vi "Initialize.vi"(6 "Serial Configuration":T1={"Baud Rate"=9600, "Parity"=0, "Data Bits"=8, "Stop Bits"=10, "Flow Control"=0} {"Flow Control" items=["None", "XON/XOFF", "RTS/CTS", "XON/XOFF & RTS/CTS", "DTR/DSR", "XON/XOFF & DTR/DSR"]; "Stop Bits" items=["1.0"=10, "1.5"=15, "2.0"=20]; "Data Bits" items=["7"=7, "8"=8]; "Parity" items=["None", "Odd", "Even", "Mark", "Space"]; "Baud Rate" items=["300"=300, "600"=600, "1200"=1200, "2400"=2400, "4800"=4800, "9600"=9600, "19200"=19200]}, 7 "error in (no error)":errorcluster, 8 "ID Query (T: Check)":bool=TRUE, 9 "VISA resource name":refnum<visa-resource-name>="TCPIP0::169.254.213.32::inst0::INSTR", 10 "BH Druck PACE Series in":refnum<class "BH Druck PACE Series.lvclass">) -> (0 "error out":errorcluster, 3 "BH Druck PACE Series out":refnum<class "BH Druck PACE Series.lvclass">)   [LabVIEW 2022 SP3, in "BH Druck PACE Series.lvclass"]
uses:
  BH Druck PACE Series.lvclass
  BH Druck PACE Series.lvclass/BH Druck PACE Series.ctl
panel:
  out "VISA resource name out":refnum<visa-resource-name>
  # "2010-2022 BH Druck Ltd.  ALL RIGHTS RESERVED."
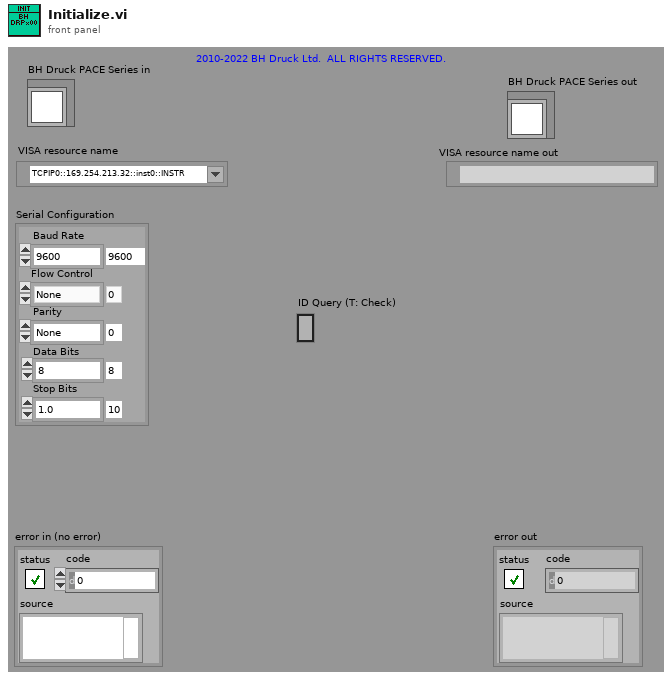
[diagram p1: front panel]
types:
  T1 = cluster{"Baud Rate":u32, "Parity":u16, "Data Bits":u16, "Stop Bits":u16, "Flow Control":u16}
  T2 = cluster{"status":bool, "code":i32, "VI name":string}
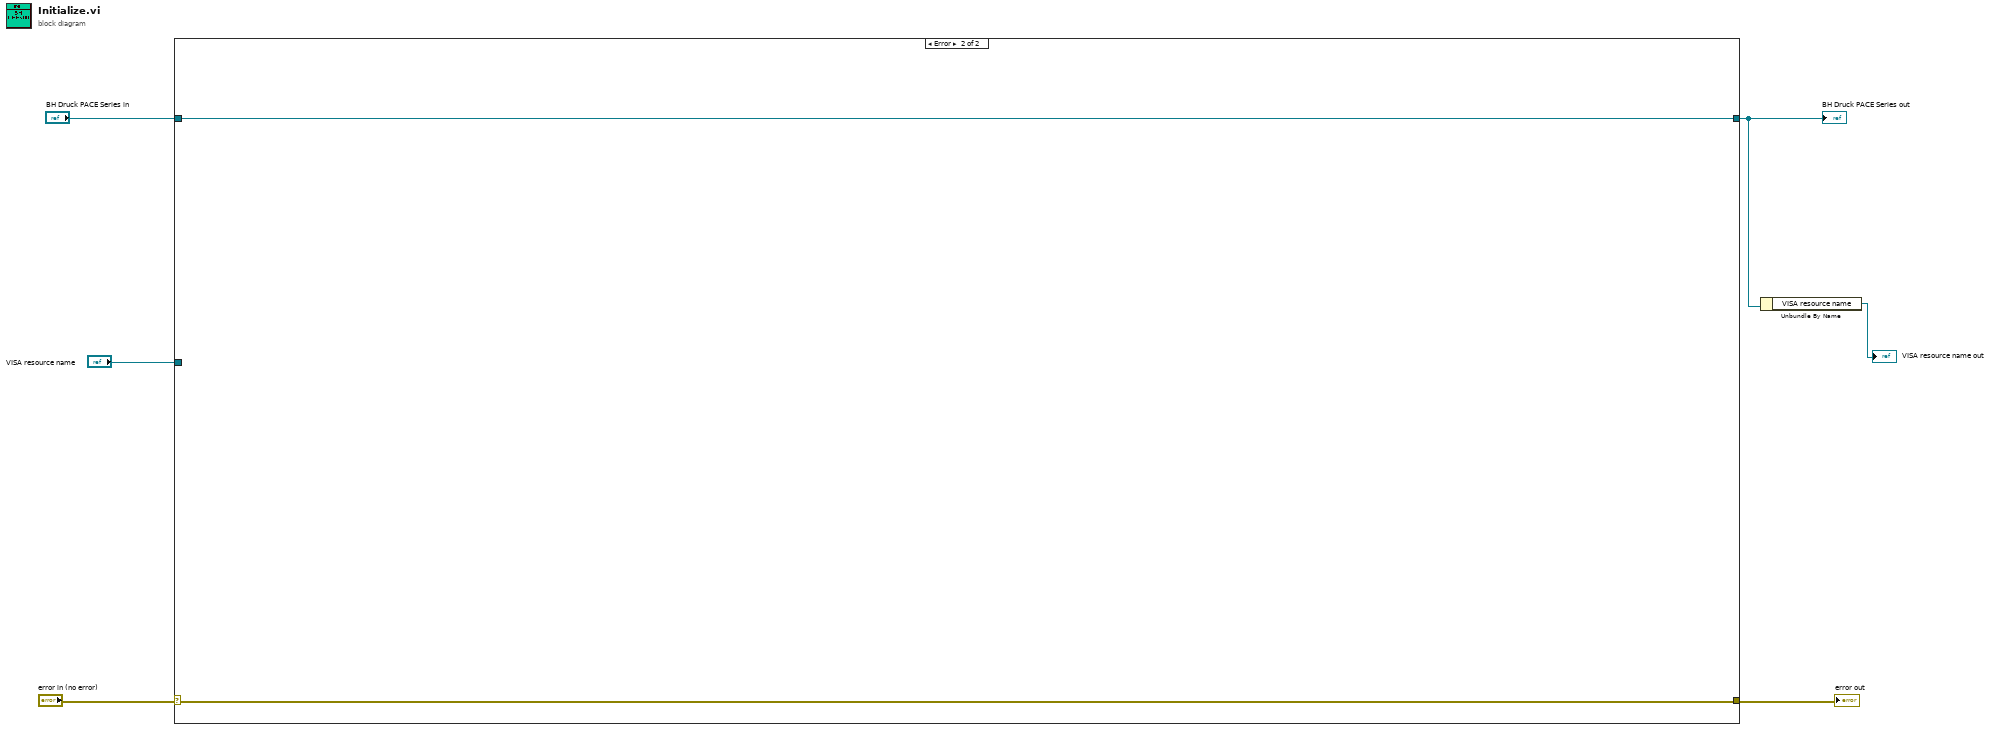
[diagram p0: block diagram]
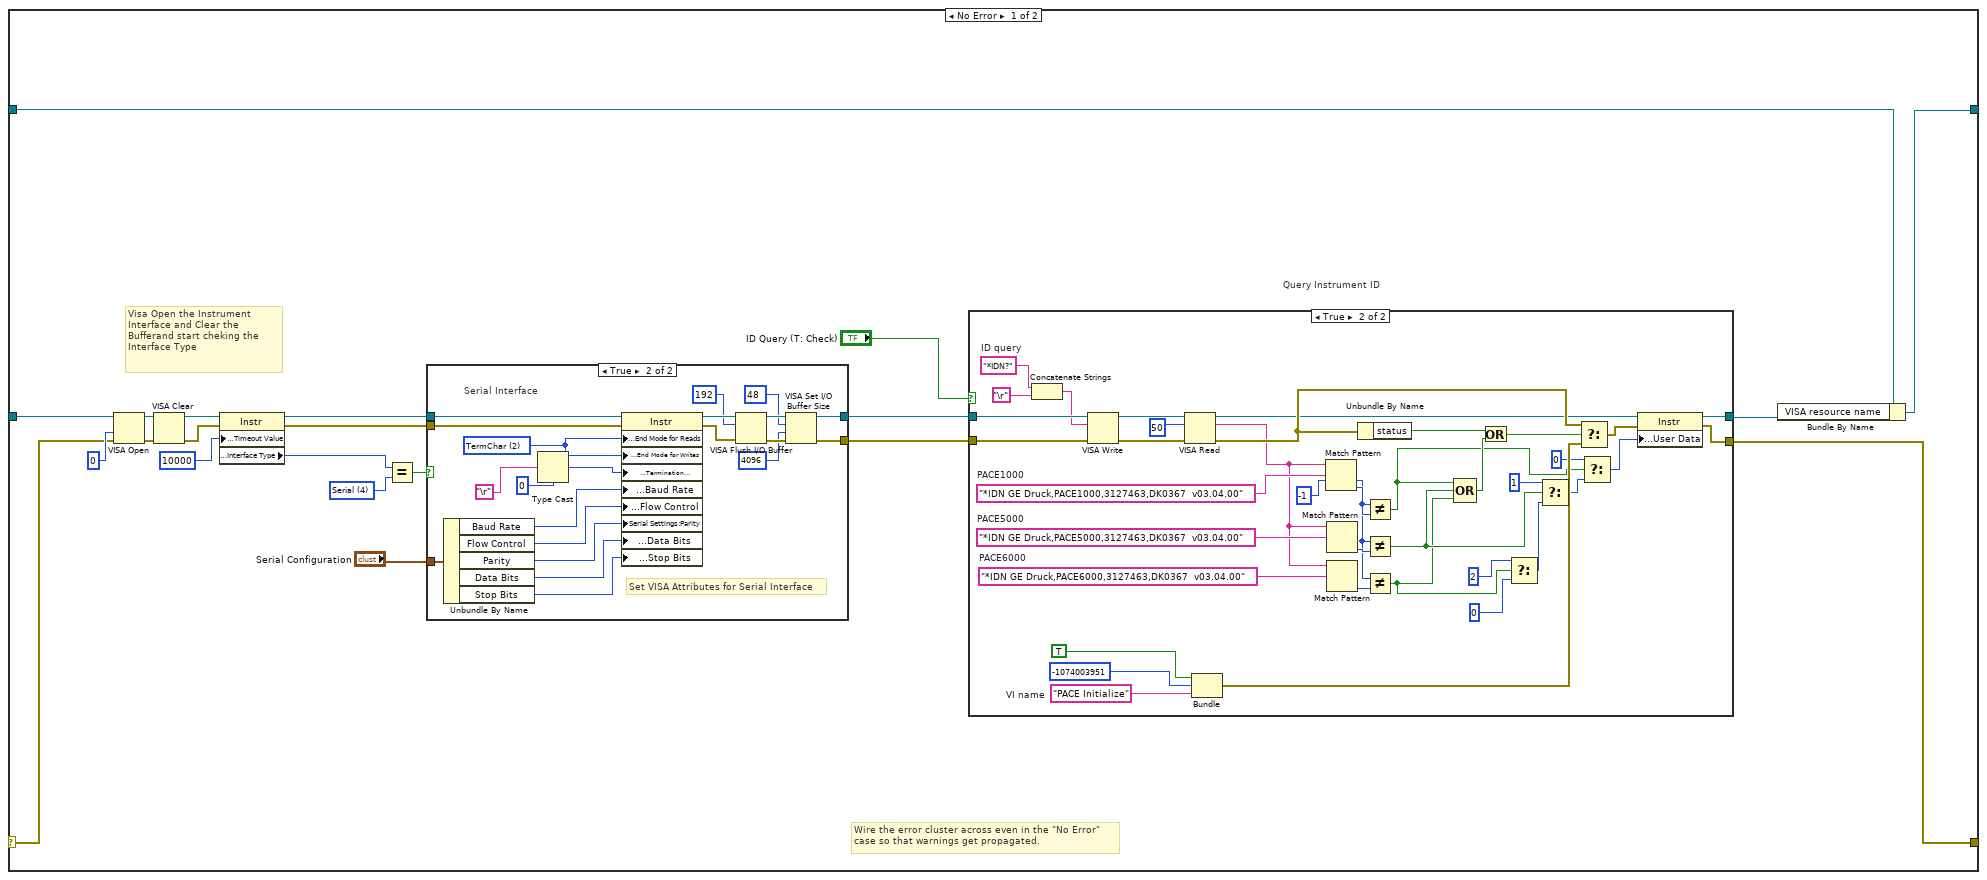
[diagram p2: hidden frame]
diagram:
  n1 = case shown="Error" "error in (no error)" {
    selector: "error in (no error)" -> [w15 w92]
    tunnel: [w8 w92] -> w5
    tunnel: [w7 w91] -> w2
    tunnel: "BH Druck PACE Series in" -> [w14 w91]
    tunnel: "VISA resource name" -> [w13 _]
    frame No Error {
      w22 = u16 4 items=["GPIB"=1, "VXI"=2, "GPIB-VXI"=3, "Serial"=4, "PXI"=5, "TCPIP"=6, "USB"=7] ("Interface Information:Interface Type")
      # "Visa Open the Instrument  Interface and Clear the Bufferand start cheking the \nInterface Type"
      # "Query Instrument ID"
      # "Wire the error cluster across even in the \"No Error\"\ncase so that warnings get propagated."
      n2 = VISA Open(access mode=u32 0, error in (no error)=w15, VISA resource name=w13) -> (VISA resource name=w20:refnum<visa-resource-name>, error out=w19:errorcluster)  [unwired: 2 in]
      n3 = VISA Clear(VISA resource name=w20, error in (no error)=w19) -> (VISA resource name out=w18:refnum<visa-resource-name>, error out=w17:errorcluster)
      n4 = property on="Property Node" class="Instr"(reference=w18, error in=w17, "General Settings:Timeout Value"=u32 10000) -> (reference out=w25:refnum<visa-resource-name>, error out=w24:errorcluster, "Interface Information:Interface Type"=w27:u16)
      n5 = Equal?(x=w27, y=w22) -> (x = y?=w23:bool)
      n6 = case shown="True" w23 {
        tunnel: [w68 w87] -> w11
        tunnel: [w69 w84] -> w10
        tunnel: w25 -> [w68 w89]
        tunnel: w24 -> [w69 w90]
        tunnel: "Serial Configuration" -> [_ w71]
        frame False {
          # "This Case Executes for GPIB ,VXI-11,TCP/IP ans Hislip Interface"
        }
        frame True {
          w78 = u16 2 items=["None", "LastBit", "TermChar"] ("Serial Settings:Serial End Mode for Reads")
          # "Set VISA Attributes for Serial Interface"
          # "Serial Interface"
          n7 = Unbundle By Name(w71) -> ("Baud Rate"=w76:u32, "Flow Control"=w73:u16, "Parity"=w74:u16, "Data Bits"=w75:u16, "Stop Bits"=w72:u16)
          n8 = Type Cast(type=u8 0, x="\r" ("Carriage Return Constant")) -> (*(type *) &x=w77:u8)
          n9 = property on="Property Node" class="Instr"(reference=w89, error in=w90, "Serial Settings:End Mode for Reads"=w78, "Serial Settings:End Mode for Writes"=w78, "Message Based Settings:Termination Character"=w77, "Serial Settings:Baud Rate"=w76, "Serial Settings:Flow Control"=w73, "Serial Settings:Parity"=w74, "Serial Settings:Data Bits"=w75, "Serial Settings:Stop Bits"=w72) -> (reference out=w83:refnum<visa-resource-name>, error out=w86:errorcluster)
          n10 = VISA Flush I/O Buffer(VISA resource name=w83, mask (16)=u16 192, error in (no error)=w86) -> (VISA resource name out=w88:refnum<visa-resource-name>, error out=w85:errorcluster)
          n11 = VISA Set I/O Buffer Size(VISA resource name=w88, mask (16)=u16 48, size (4096)=u32 4096 ("size (0)"), error in (no error)=w85) -> (VISA resource name out=w87:refnum<visa-resource-name>, error out=w84:errorcluster)
        }
      }
      n12 = case shown="True" "ID Query (T: Check)" {
        tunnel: [w28 w43] -> w8
        tunnel: [w29 w44] -> w9
        tunnel: w11 -> [w29 w63]
        tunnel: w10 -> [w28 w62]
        frame False {
        }
        frame True {
          w51 = "*IDN GE Druck,PACE6000,3127463,DK0367  v03.04.00"  # PACE6000
          w53 = "*IDN GE Druck,PACE5000,3127463,DK0367  v03.04.00"  # PACE5000
          w54 = "*IDN GE Druck,PACE1000,3127463,DK0367  v03.04.00"  # PACE1000
          w59 = "PACE Initialize"  # VI name
          w48 = -1
          w32 = "*IDN?"  # ID query
          n13 = Concatenate Strings(w32, "\r") -> (w30:string)
          n14 = VISA Write(VISA resource name=w63, write buffer=w30, error in (no error)=w62) -> (VISA resource name out=w64:refnum<visa-resource-name>, error out=w67:errorcluster)  [unwired: 1 out]
          n15 = VISA Read(VISA resource name=w64, byte count=u32 50, error in (no error)=w67) -> (VISA resource name out=w46:refnum<visa-resource-name>, read buffer=w49:string, error out=w56:errorcluster)  [unwired: 1 out]
          n16 = Bundle(TRUE, -1074003951, "VI name"=w59) -> (w65:cluster{bool, i32, "VI name":string})  [unwired: 1 in]
          n17 = Match Pattern(string=w49, regular expression=w54) -> (offset past match=w60:i32)  [unwired: 1 in, 3 out]
          n18 = Match Pattern(string=w49, regular expression=w53) -> (offset past match=w52:i32)  [unwired: 1 in, 3 out]
          n19 = Match Pattern(string=w49, regular expression=w51) -> (offset past match=w50:i32)  [unwired: 1 in, 3 out]
          n20 = Unbundle By Name(w56) -> ("status"=w55:bool)
          n21 = Not Equal?(x=w48, y=w60) -> (x != y?=w36:bool)
          n22 = Not Equal?(x=w48, y=w52) -> (x != y?=w42:bool)
          n23 = Not Equal?(x=w48, y=w50) -> (x != y?=w41:bool)
          n24 = Compound Arithmetic op=OR(w36, w42, w41) -> (w47:bool)
          n25 = Or(x=w55, y=w47) -> (x .or. y?=w57:bool)
          n26 = Select(t=u32 2, s=w41, f=u32 0) -> (s? t:f=w38:u32)
          n27 = Select(t=u32 1, s=w42, f=w38) -> (s? t:f=w35:u32)
          n28 = Select(t=w56, s=w57, f=w65) -> (s? t:f=w45:T2)
          n29 = Select(t=u32 0, s=w36, f=w35) -> (s? t:f=w33:u32)
          n30 = property class="Instr"(reference=w46, error in=w45, "General Settings:User Data"=w33) -> (reference out=w44:refnum<visa-resource-name>, error out=w43:errorcluster)
        }
      }
      n31 = Bundle By Name(cluster=w14, "VISA resource name"=w9) -> (w7:refnum<class "BH Druck PACE Series.lvclass">)
    }
    frame Error {
    }
  }
  "error out" <- w5
  "BH Druck PACE Series out" <- w2
  n32 = Unbundle By Name(w2) -> ("VISA resource name"=→"VISA resource name out":refnum<visa-resource-name>)
